vi "Gaussian_process.vi"   [LabVIEW 2020]
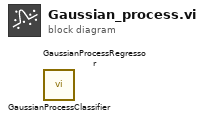
[diagram p0: block diagram]
diagram:
  n1 = call "GaussianProcessClassifier.vi"() -> ()  [unwired: 10 in, 2 out]
  n2 = call "GaussianProcessRegressor.vi"() -> ()  [unwired: 10 in, 2 out]
